vi "KepcoDCPwr Current Software Timed Ramp Example.vi"(0 "VISA resource name":refnum<visa-resource-name>="BOP", 2 "OPpen/Close":bool=TRUE, 5 "Model In":string, 11 "error in (no error)":errorcluster) -> (8 "actual current":dbl, 15 "error out":errorcluster)   [LabVIEW 2013]
panel:
  in  "Ramp Direction":bool
  out "Current vs Time":cluster{dbl[], dbl[]}(graph)={[0.0, 50.0, 100.0, 150.0, 200.0, 250.0, 300.0, 350.0, 400.0, 450.0, 500.0], [10.0, 9.0, 8.0, 7.0, 6.0, 5.0, 4.0, 3.0, 2.0, 1.0, 0.0]}
  in  "Stop":bool
  in  "Readback Current":bool
  in  "Readback Voltage":bool
  in  "Start Ramp":bool
  in  "Current Increment":dbl=1.0 step=1e-05 format="%.6f"
  in  "Dwell (ms)":u32=50 max=5000 step=1
  in  "End (Current)":dbl=10.0 format="%.2f"
  in  "Start (Current)":ext format="%.2f"
  in  "# of Cycles":i32=100
  in  "Repeat":bool=TRUE
  in  "Disable @ End":bool
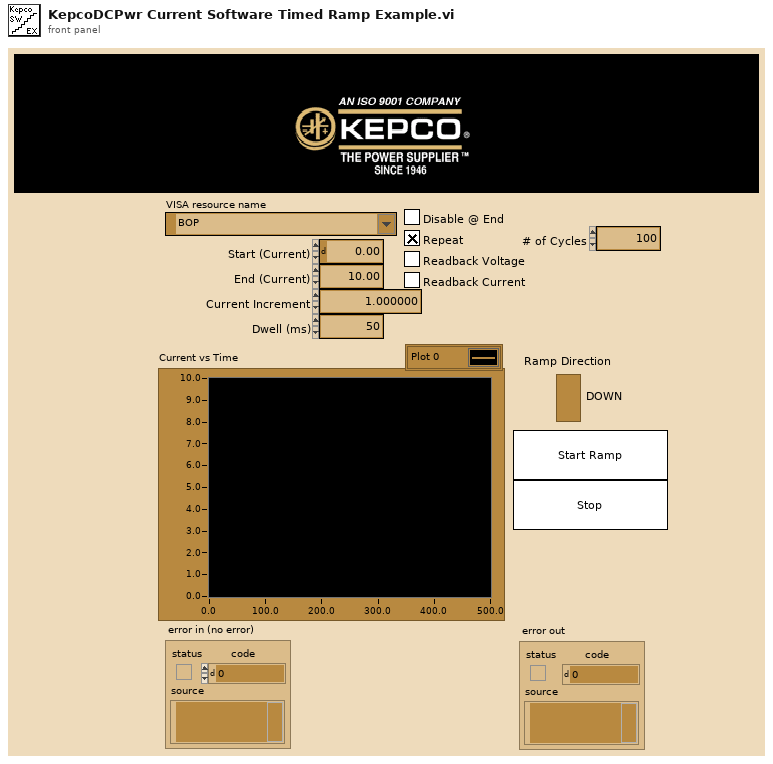
[diagram p1: front panel]
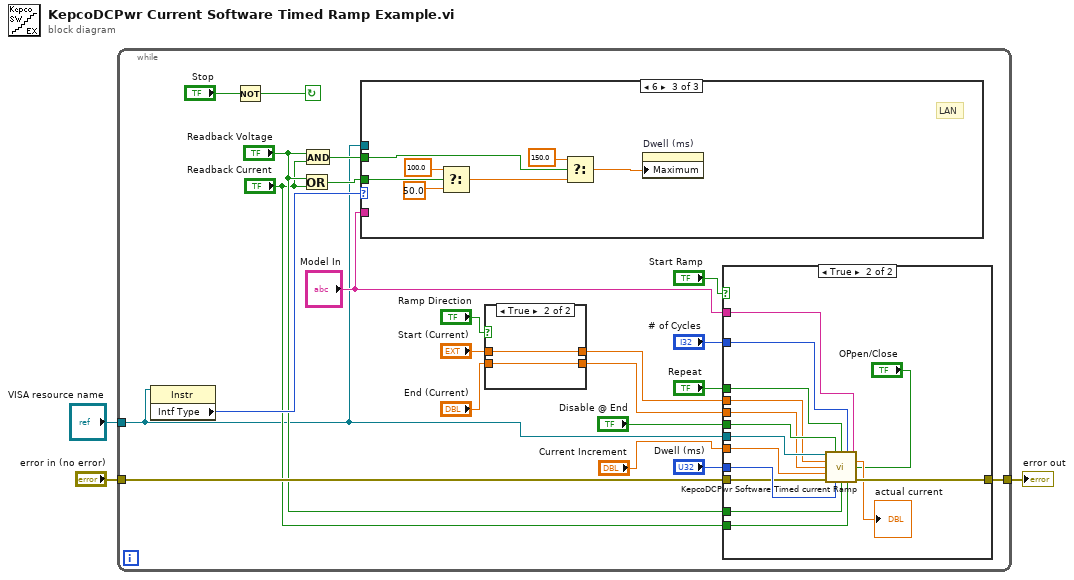
[diagram p0: block diagram]
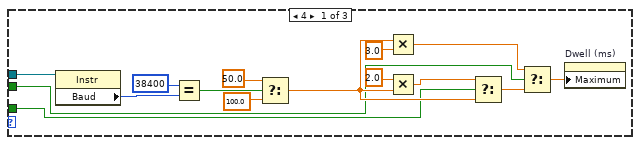
[diagram p2: hidden frame]
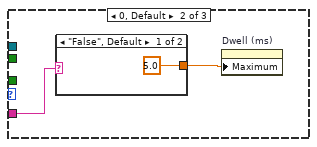
[diagram p3: hidden frame]
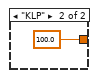
[diagram p4: hidden frame]
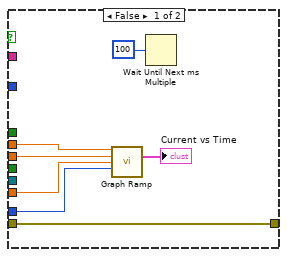
[diagram p5: hidden frame]
diagram:
  n1 = while {
    tunnel: "VISA resource name" -> [w4]
    tunnel: [w24] -> w2
    tunnel: "error in (no error)" -> [w25]
    stop <- w13 continue-if-true
    n2 = property class="Instr"(reference=w4) -> ("Intf Type"=w10:u16)  [unwired: 1 in, 2 out]
    n3 = Not(x="Stop") -> (.not. x?=w13:bool)
    n4 = Or(x="Readback Voltage", y="Readback Current") -> (x .or. y?=w5:bool)
    n5 = And(x="Readback Voltage", y="Readback Current") -> (x .and. y?=w6:bool)
    n6 = case shown="6" w10 {
      tunnel: "Model In" -> [_ w42 _]
      tunnel: w6 -> [w27 _ w46]
      tunnel: w5 -> [w28 _ w45]
      tunnel: w4 -> [w26 _ _]
      frame 4 {
        n7 = property class="Instr"(reference=w26) -> ("Baud"=w34:u32)  [unwired: 1 in, 2 out]
        n8 = Equal?(x=u32 38400, y=w34) -> (x = y?=w33:bool)
        n9 = Select(t=50.0 ("f"), s=w33, f=100.0) -> (s? t:f=w30:dbl)
        n10 = Multiply(x=w30, y=3.0) -> (x*y=w37:dbl)
        n11 = Multiply(x=2.0, y=w30) -> (x*y=w36:dbl)
        n12 = Select(t=w36, s=w28, f=w30) -> (s? t:f=w40:dbl)
        n13 = Select(t=w37, s=w27, f=w40) -> (s? t:f=w29:dbl)
        n14 = property on="Dwell (ms)" class="DigNum (strict)"("Maximum"=w29) -> ()  [unwired: 2 in, 2 out]
      }
      frame 0, Default {
        n15 = case shown="\"False\", Default" w42 {
          tunnel: [5.0 ("Data Entry Limits:Maximum") 100.0 ("Data Entry Limits:Maximum")] -> w41
          frame "False", Default {
          }
          frame "KLP" {
          }
        }
        n16 = property on="Dwell (ms)" class="DigNum (strict)"("Maximum"=w41) -> ()  [unwired: 2 in, 2 out]
      }
      frame 6 {
        # "LAN"
        n17 = Select(t=100.0, s=w45, f=50.0) -> (s? t:f=w51:dbl)
        n18 = Select(t=150.0, s=w46, f=w51) -> (s? t:f=w47:dbl)
        n19 = property on="Dwell (ms)" class="DigNum (strict)"("Maximum"=w47) -> ()  [unwired: 2 in, 2 out]
      }
    }
    n20 = case shown="True" "Ramp Direction" {
      tunnel: "End (Current)" -> [w75 w76]
      tunnel: "Start (Current)" -> [w74 w77]
      tunnel: [w75 w77] -> w16
      tunnel: [w74 w76] -> w15
      frame False {
      }
      frame True {
      }
    }
    n21 = case shown="True" "Start Ramp" {
      tunnel: w25 -> [w58 w62]
      tunnel: [w58 w72] -> w24
      tunnel: "Dwell (ms)" -> [w53 w65]
      tunnel: "Current Increment" -> [w54 w66]
      tunnel: "Readback Current" -> [_ w63]
      tunnel: "Readback Voltage" -> [_ w64]
      tunnel: "Disable @ End" -> [_ w70]
      tunnel: "Repeat" -> [_ w71]
      tunnel: "# of Cycles" -> [_ w73]
      tunnel: w16 -> [w56 w68]
      tunnel: w15 -> [w55 w67]
      tunnel: w4 -> [_ w69]
      tunnel: "Model In" -> [_ w59]
      frame False {
        n22 = call "Graph Ramp.vi"("Start (Volts)"=w56, "End (volts)"=w55, "Voltage Increment"=w54, "Dwell (sec)"=w53) -> ("Voltage vs Time"=→"Current vs Time":cluster{dbl[], dbl[]})  [unwired: 11 out]
        n23 = Wait Until Next ms Multiple(millisecond multiple=u32 100) -> ()  [unwired: 1 out]
      }
      frame True {
        n24 = call "KepcoDCPwr Software Timed current Ramp.vi"("VISA resource name"=w69, "Disable @ End"=w70, "Repeat"=w71, "# of Cycles"=w73, "Model In"=w59, "Start (current)"=w68, "End (current)"=w67, "OPpen/Close"="OPpen/Close", "current Increment"=w66, "error in (no error)"=w62, "Dwell (ms)"=w65, "Readback Voltage"=w64, "Readback Current"=w63) -> ("actual current"=→"actual current":dbl, "error out"=w72:errorcluster)  [unwired: 1 out]
      }
    }
  }
  "error out" <- w2
